vi "Example3.vi"() -> ()   [LabVIEW 2020, in "LcPictureBox.lvclass"]
uses:
  <userlib>/_LabVIEWCommon/LcPictureBox_class/LcPictureBox.lvclass
  System.Windows.Forms
  <userlib>/_LabVIEWCommon/LcPictureBox_class/Pen.ctl
  <userlib>/_LabVIEWCommon/LcPictureBox_class/SmoothingMode.ctl
panel:
  in  "PictureBox 1":refnum<k24>(container)
  in  "PictureBox 2":refnum<k24>(container)
  out "error out 2":errorcluster
  out "error out":errorcluster
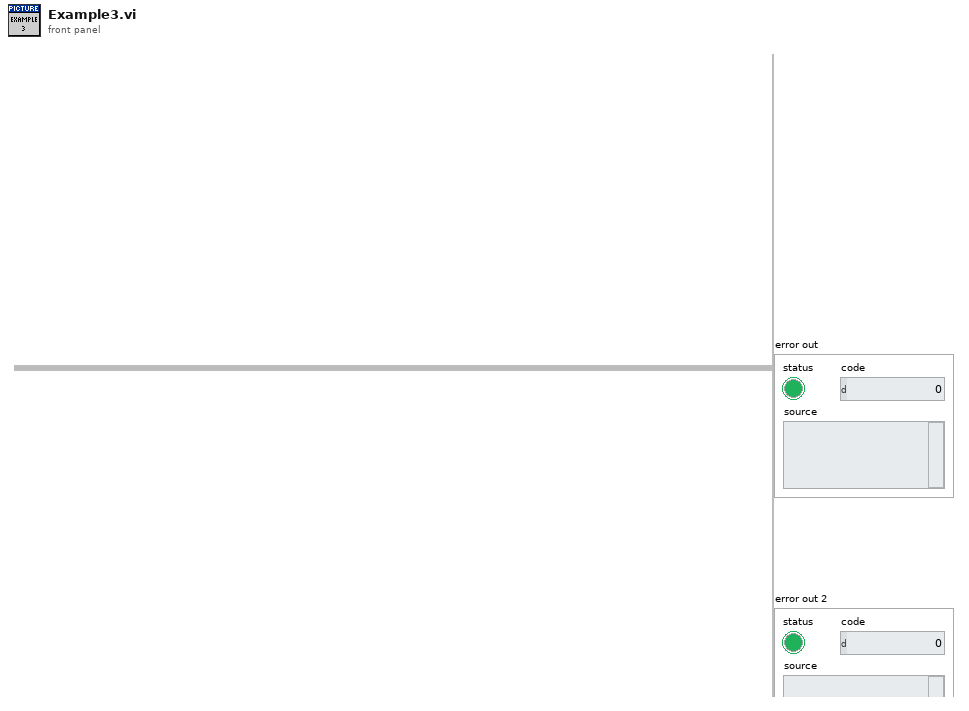
[diagram p1: front panel]
types:
  T1 = typedef "LcPictureBox.lvclass/Pen.ctl" = cluster{"Width":dbl, "Style":enum32{"Solid", "Dash", "Dot", "DashDot", "DashDotDot"}}
  T2 = typedef "LcPictureBox.lvclass/SmoothingMode.ctl" = enum16{"None", "HighSpeed", "HighQuality", "AntiAlias"}
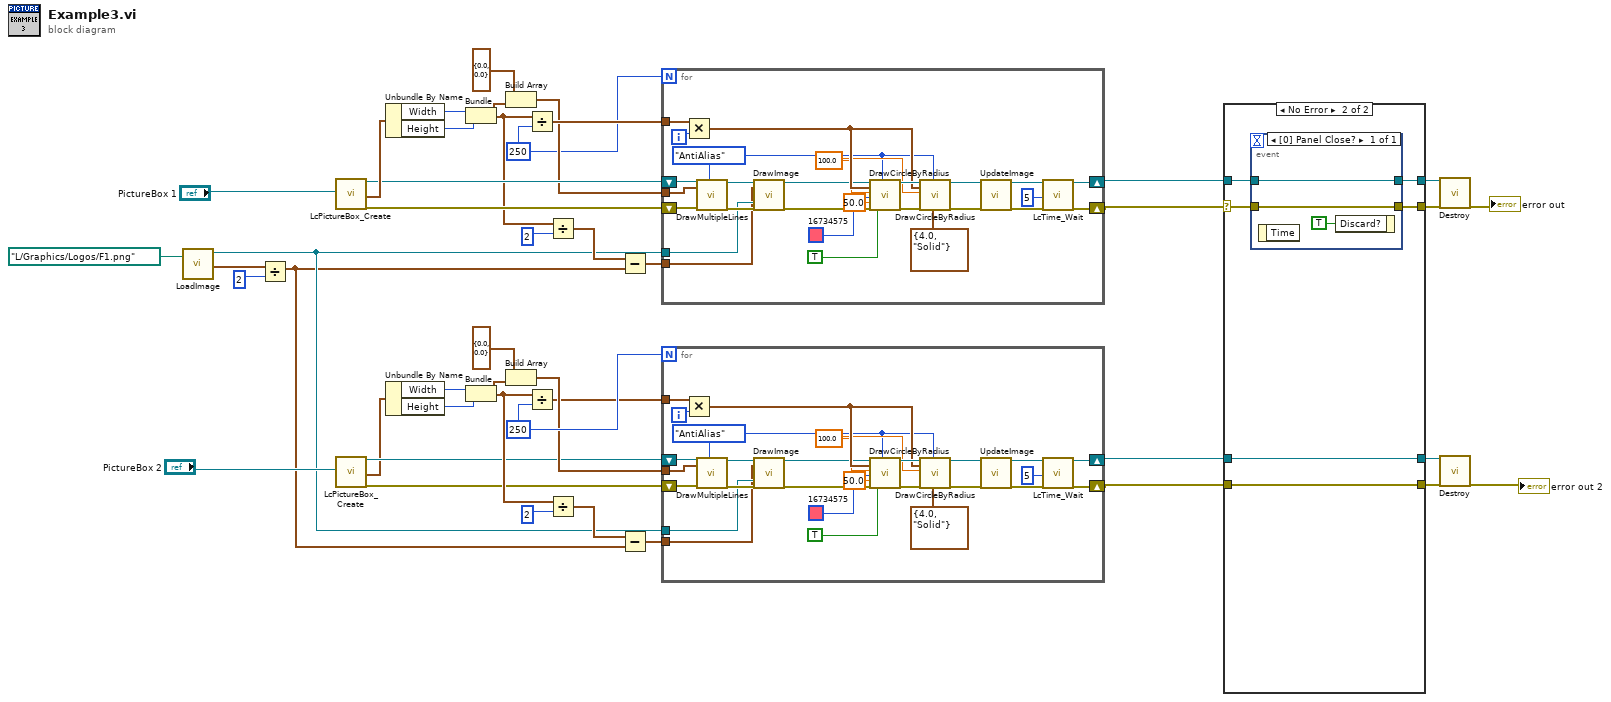
[diagram p0: block diagram]
diagram:
  w17 = 250 ("y")
  w30 = 250 ("y")
  n1 = call <userlib>:"LoadImage.vi"("ImageFile"=path "L:/Graphics/Logos/F1.png" ("Filename")) -> ("ImageOut"=w2:refnum<k24>, "ImageSize"=w27:cluster{"Width":i32, "Height":i32})  [unwired: 16 in, 1 out]
  n2 = Divide(x=w27, y=2) -> (x/y=w1:cluster{"Width":dbl, "Height":dbl})
  n3 = call <userlib>:"LcPictureBox_Create.vi"("PictureBox"="PictureBox 1") -> ("reference out"=w33:refnum<class "LcPictureBox.lvclass">, "ImageSizeUsed"=w43:cluster{"Width":i32, "Height":i32}, "Error Out"=w31:errorcluster)  [unwired: 16 in]
  n4 = call <userlib>:"LcPictureBox_Create.vi"("PictureBox"="PictureBox 2") -> ("reference out"=w14:refnum<class "LcPictureBox.lvclass">, "ImageSizeUsed"=w9:cluster{"Width":i32, "Height":i32}, "Error Out"=w16:errorcluster)  [unwired: 16 in]
  n5 = Unbundle By Name(w43) -> ("Width"=w37:i32, "Height"=w36:i32)
  n6 = Unbundle By Name(w9) -> ("Width"=w10:i32, "Height"=w11:i32)
  n7 = Bundle("Width"=w37, "Height"=w36) -> (w24:cluster{"Width":i32, "Height":i32})  [unwired: 1 in]
  n8 = Bundle("Width"=w10, "Height"=w11) -> (w19:cluster{"Width":i32, "Height":i32})  [unwired: 1 in]
  n9 = Build Array(cluster{"x":dbl, "y":dbl} {"x"=0.0, "y"=0.0} ("Point"), w24) -> (w32:cluster{"x":dbl, "y":dbl}[])
  n10 = Build Array(cluster{"x":dbl, "y":dbl} {"x"=0.0, "y"=0.0} ("Point"), w19) -> (w15:cluster{"x":dbl, "y":dbl}[])
  n11 = Divide(x=w24, y=w30) -> (x/y=w34:cluster{"Width":dbl, "Height":dbl})
  n12 = Divide(x=w19, y=w17) -> (x/y=w13:cluster{"Width":dbl, "Height":dbl})
  n13 = Divide(x=w24, y=2) -> (x/y=w23:cluster{"Width":dbl, "Height":dbl})
  n14 = Divide(x=w19, y=2) -> (x/y=w20:cluster{"Width":dbl, "Height":dbl})
  n15 = Subtract(x=w23, y=w1) -> (x-y=w22:cluster{"Width":dbl, "Height":dbl})
  n16 = Subtract(x=w20, y=w1) -> (x-y=w21:cluster{"Width":dbl, "Height":dbl})
  n17 = for {
    N: w30 -> [_]
    tunnel: w34 -> [w69]
    tunnel: w32 -> [w66]
    shift-right: [w62] -> w28
    shift-left: w31 -> [w65]
    shift-right: [w61] -> w29
    shift-left: w33 -> [w67]
    tunnel: w2 -> [w46]
    tunnel: w22 -> [w45]
    i -> [w68]
    w44 = SmoothingMode."AntiAlias" ("SmoothingMode")
    w51 = sgl 100.0 ("Radius")
    n18 = Multiply(x=w69, y=w68) -> (x*y=w52:cluster{"Width":dbl, "Height":dbl})
    n19 = call-dynamic "DrawMultipleLines.vi"("reference in"=w67, "LineEndPoints"=w66, "Error In"=w65, "SmoothingMode"=w44) -> ("reference out"=w50:refnum<class "LcPictureBox.lvclass">, "Error Out"=w49:errorcluster)  [unwired: 14 in]
    n20 = call-dynamic "DrawImage.vi"("reference in"=w50, "UpperLeftCorner"=w45, "Image"=w46, "Error In"=w49) -> ("reference out"=w48:refnum<class "LcPictureBox.lvclass">, "Error Out"=w47:errorcluster)  [unwired: 14 in]
    n21 = call-dynamic "DrawCircleByRadius.vi"("reference in"=w48, "Center"=w52, "Radius"=w51, "Color(Black)"=u32 16734575, "Alpha(100%)"=50.0, "Error In"=w47, "Fill(False)"=TRUE, "SmoothingMode"=w44) -> ("reference out"=w57:refnum<class "LcPictureBox.lvclass">, "Error Out"=w55:errorcluster)  [unwired: 10 in]
    n22 = call-dynamic "DrawCircleByRadius.vi"("reference in"=w57, "Center"=w52, "Radius"=w51, "Error In"=w55, "SmoothingMode"=w44, "Pen(Width=1, Solid)"=T1 {"Width"=4.0, "Style"=enum."Solid"}) -> ("reference out"=w56:refnum<class "LcPictureBox.lvclass">, "Error Out"=w54:errorcluster)  [unwired: 12 in]
    n23 = call-dynamic "UpdateImage.vi"("reference in"=w56, "Error In"=w54) -> ("reference out"=w61:refnum<class "LcPictureBox.lvclass">, "Error Out"=w64:errorcluster)  [unwired: 14 in, 2 out]
    n24 = call <userlib>:"LcTime_Wait.vi"("msToWait"=u32 5, "error in (no error)"=w64) -> ("error out"=w62:errorcluster)  [unwired: 15 in, 2 out]
  }
  n25 = for {
    N: w17 -> [_]
    tunnel: w13 -> [w95]
    tunnel: w15 -> [w92]
    shift-right: [w88] -> w5
    shift-left: w16 -> [w91]
    shift-right: [w87] -> w7
    shift-left: w14 -> [w93]
    tunnel: w2 -> [w72]
    tunnel: w21 -> [w71]
    i -> [w94]
    w70 = SmoothingMode."AntiAlias" ("SmoothingMode")
    w77 = sgl 100.0 ("Radius")
    n26 = Multiply(x=w95, y=w94) -> (x*y=w78:cluster{"Width":dbl, "Height":dbl})
    n27 = call-dynamic "DrawMultipleLines.vi"("reference in"=w93, "LineEndPoints"=w92, "Error In"=w91, "SmoothingMode"=w70) -> ("reference out"=w76:refnum<class "LcPictureBox.lvclass">, "Error Out"=w75:errorcluster)  [unwired: 14 in]
    n28 = call-dynamic "DrawImage.vi"("reference in"=w76, "UpperLeftCorner"=w71, "Image"=w72, "Error In"=w75) -> ("reference out"=w74:refnum<class "LcPictureBox.lvclass">, "Error Out"=w73:errorcluster)  [unwired: 14 in]
    n29 = call-dynamic "DrawCircleByRadius.vi"("reference in"=w74, "Center"=w78, "Radius"=w77, "Color(Black)"=u32 16734575, "Alpha(100%)"=50.0, "Error In"=w73, "Fill(False)"=TRUE, "SmoothingMode"=w70) -> ("reference out"=w83:refnum<class "LcPictureBox.lvclass">, "Error Out"=w81:errorcluster)  [unwired: 10 in]
    n30 = call-dynamic "DrawCircleByRadius.vi"("reference in"=w83, "Center"=w78, "Radius"=w77, "Error In"=w81, "SmoothingMode"=w70, "Pen(Width=1, Solid)"=T1 {"Width"=4.0, "Style"=enum."Solid"}) -> ("reference out"=w82:refnum<class "LcPictureBox.lvclass">, "Error Out"=w80:errorcluster)  [unwired: 12 in]
    n31 = call-dynamic "UpdateImage.vi"("reference in"=w82, "Error In"=w80) -> ("reference out"=w87:refnum<class "LcPictureBox.lvclass">, "Error Out"=w90:errorcluster)  [unwired: 14 in, 2 out]
    n32 = call <userlib>:"LcTime_Wait.vi"("msToWait"=u32 5, "error in (no error)"=w90) -> ("error out"=w88:errorcluster)  [unwired: 15 in, 2 out]
  }
  n33 = case shown="No Error" w28 {
    selector: w28 -> [w99 w102]
    tunnel: [w99 w105] -> w40
    tunnel: w29 -> [w98 w104]
    tunnel: [w98 w103] -> w39
    tunnel: w7 -> [w97 w101]
    tunnel: [w97 w101] -> w6
    tunnel: w5 -> [w96 w100]
    tunnel: [w96 w100] -> w4
    frame Error {
    }
    frame No Error {
      n34 = event shown="[0] Panel Close?" {
        selector: _ -> [_]
        dyn-events: _ -> [_]
        timeout: _ -> [_]
        tunnel: w102 -> [w107]
        tunnel: [w107] -> w105
        tunnel: w104 -> [w106]
        tunnel: [w106] -> w103
        event Panel Close? {
          n35 = event-data() -> ()  [unwired: 1 in, 1 out]
          n36 = event-data("Discard?"=TRUE) -> ()  [unwired: 1 in, 1 out]
        }
      }
    }
  }
  n37 = call-dynamic "Destroy.vi"("reference in"=w39, "Error In"=w40) -> ("Error Out"=→"error out":errorcluster)  [unwired: 16 in, 1 out]
  n38 = call-dynamic "Destroy.vi"("reference in"=w6, "Error In"=w4) -> ("Error Out"=→"error out 2":errorcluster)  [unwired: 16 in, 1 out]
